vi "Set Initialize.vi"(8 "error in (no error)":errorcluster, 10 "Initialize":bool, 11 "Abstract Initialize Msg in":refnum<class "Abstract Initialize Msg.lvclass">) -> (0 "error out":errorcluster, 3 "Abstract Initialize Msg out":refnum<class "Abstract Initialize Msg.lvclass">)   [LabVIEW 2013, in "Create Project Model.lvlib" / "Abstract Initialize Msg.lvclass"]
uses:
  Abstract Initialize Msg.lvclass
  Abstract Initialize Msg.lvclass/Abstract Initialize Msg.ctl
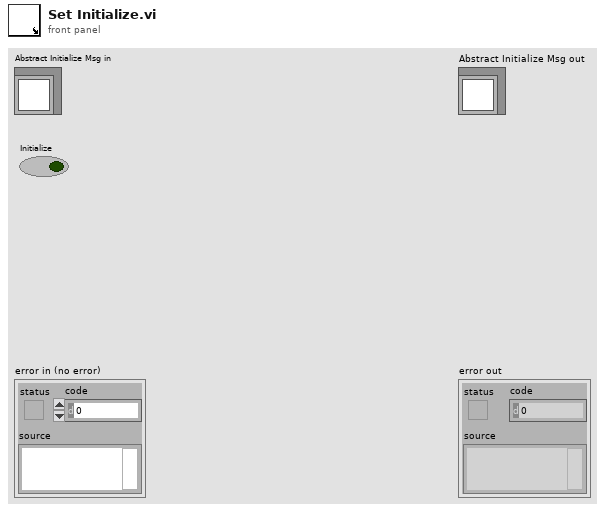
[diagram p1: front panel]
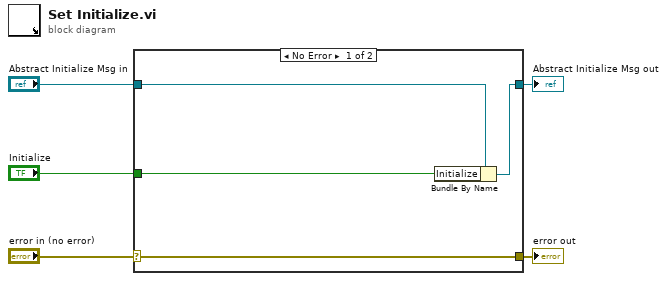
[diagram p0: block diagram]
diagram:
  n1 = case shown="No Error" "error in (no error)" {
    selector: "error in (no error)" -> [w9 w10]
    tunnel: [w9 w10] -> w4
    tunnel: [w7 w11] -> w2
    tunnel: "Abstract Initialize Msg in" -> [w8 w11]
    tunnel: "Initialize" -> [w6 _]
    frame No Error {
      n2 = Bundle By Name(cluster=w8, "Initialize"=w6) -> (w7:refnum<class "Abstract Initialize Msg.lvclass">)
    }
    frame Error {
    }
  }
  "error out" <- w4
  "Abstract Initialize Msg out" <- w2
